vi "DETECTION REPORT for manual.vi"(7 "NEW PARAMETERS":T1, 8 "error in (no error)":errorcluster, 9 "return value 3":cluster{"major":dbl, "minor":dbl, "average":dbl}, 10 "Image File Path":path, 11 "Main Ref":T2) -> (0 "error out":errorcluster)   [LabVIEW 2025]
uses:
  <vilib>/Exaprom PDF/Controls/Font Controls/Font complete cluster.ctl
  <vilib>/Exaprom PDF/Controls/Font Controls/Font size.ctl
  <vilib>/Exaprom PDF/Controls/Font Controls/Font color.ctl
  <vilib>/Exaprom PDF/Controls/Font Controls/Type and encoding.ctl
  <vilib>/Exaprom PDF/Controls/Text Controls/Unicode/Type and run direction.ctl
  <vilib>/Exaprom PDF/Controls/Header, Footer and Watermark Controls/Header or Footer  Text cluster.ctl
  <vilib>/Exaprom PDF/Controls/Table Controls/Cell Alignment 20px.ctl
  <vilib>/Exaprom PDF/Controls/Text Controls/Line spacing.ctl
  <vilib>/Exaprom PDF/Controls/Font Controls/Font complete cluster horizontal.ctl
  <vilib>/Exaprom PDF/Controls/Header, Footer and Watermark Controls/Header or Footer Line cluster.ctl
  <vilib>/Exaprom PDF/Controls/Header, Footer and Watermark Controls/Header Footer Line.ctl
  <vilib>/Exaprom PDF/Controls/Header, Footer and Watermark Controls/Watermark Text Cluster.ctl
  <vilib>/Exaprom PDF/Controls/Header, Footer and Watermark Controls/Watermark Position.ctl
  <vilib>/Exaprom PDF/Controls/Header, Footer and Watermark Controls/Header footer horiz alignment.ctl
  <vilib>/Exaprom PDF/Controls/Image Controls/Image alignment and position.ctl
  <vilib>/Exaprom PDF/Controls/Image Controls/Image aligment.ctl
  <vilib>/Exaprom PDF/Controls/Image Controls/Image border.ctl
  <vilib>/Exaprom PDF/Controls/Table Controls/Table properties.ctl
  <vilib>/Exaprom PDF/Controls/Table Controls/Table position.ctl
  <vilib>/Exaprom PDF/Controls/Header, Footer and Watermark Controls/Header or Footer.ctl
  <vilib>/Exaprom PDF/Controls/Header, Footer and Watermark Controls/Header or Footer  Image cluster.ctl
  <vilib>/Exaprom PDF/Controls/Table Controls/Cell Font, type, Alignment and LS V2.ctl
  <vilib>/Exaprom PDF/Controls/Table Controls/Cell Type, Alignment and LS.ctl
  <vilib>/Exaprom PDF/Controls/Table Controls/Text vertical arrangement.ctl
  <vilib>/Utility/error.llb/Trim Whitespace One-Sided.vi
  <vilib>/Exaprom PDF/VIs/Low level/Header, Footer and Watermark Low level/Append Image HF.vi
  <vilib>/Exaprom PDF/VIs/Low level/Header, Footer and Watermark Low level/Append Text HF.vi
  <vilib>/Exaprom PDF/VIs/Low level/Header, Footer and Watermark Low level/AppendLine seperator.vi
  <vilib>/Exaprom PDF/VIs/Text/Append Phrase.vi
  <vilib>/Exaprom PDF/VIs/Low level/Header, Footer and Watermark Low level/Append Watermark Text.vi
panel:
  in  "Watermark Text 2":T3={"Text "="PALTRO", "Opacity (%)"=5.0, "Position"={"Position"=enum."Center (text section)", "X"=0.0, "Y"=0.0}, "Automatic"=TRUE, "Font"={"Font Name"="", "Size"=-1.0, "Color"=0}, "Alignment"=enum."Center", "Rotate(°)"=0.0}
  in  "Footer Line 2":T8={"H/F Line"=enum."Horizontal line", "Thickness (point)"=0.75, " Colour"=7171459}
  in  "Header Line":T8={"H/F Line"=enum."Horizontal line", "Thickness (point)"=0.75, " Colour"=7171459}
  in  "Footer Text":T10={"Start at page"=1, "Cell Alignment"=4, "Line spacing"=enum."Select", "Text"="Fully automated next-gen fuel and lubricant testers: BOCLE-adv , HFRR-ADV , FBT-3-P", "Font complete"={"Name"="", "Size"=5.0, "Color"=16777224, "Style"={"Bold"=FALSE, "Italic"=FALSE, "Underline"=TRUE, "Strikeout"=FALSE}, "Type"={"Type&direction"=enum."Select", "Embedded"=FALSE, "Encoding"=""}}, "Link"="https://www.paltro.com/products/product-selector/lubricity"}
  in  "Date and Time :":string
  in  "Observations :":string
  in  "Scar Image Path :":path
  in  "Header or footer":T10={"Start at page"=1, "Cell Alignment"=4, "Line spacing"=enum."Select", "Text"="                                            ", "Font complete"={"Name"="", "Size"=-1.0, "Color"=0, "Style"={"Bold"=FALSE, "Italic"=FALSE, "Underline"=FALSE, "Strikeout"=FALSE}, "Type"={"Type&direction"=enum."Select", "Embedded"=FALSE, "Encoding"=""}}, "Link"=""}
  in  "Font":T16={"Name"="", "Size"=18.0, "Color"=0, "Style"={"Bold"=TRUE, "Italic"=FALSE, "Underline"=FALSE, "Strikeout"=FALSE}, "Type"={"Type&direction"=enum."Select", "Embedded"=FALSE, "Encoding"=""}}
  in  "Font 2":T16={"Name"="", "Size"=6.0, "Color"=0, "Style"={"Bold"=FALSE, "Italic"=TRUE, "Underline"=FALSE, "Strikeout"=FALSE}, "Type"={"Type&direction"=enum."Select", "Embedded"=FALSE, "Encoding"=""}}
  in  "File Name :":string(combo)
  out "folder names":string[](array[string])
  out "path out":path
  in  "Automated":bool
  in  "Test Method":string
  in  "Fuel Description":string
  out "Operator :":string
types:
  T1 = cluster{"Initial Humidity (%RH)":string, "Final Humidity (%RH)":string, "Initial Air Temperature (°C)":string, "Final Air Temperature (°C)":string, "Specimen Tested":string, "Remarks":string}
  T2 = cluster{"File Name":string, "Test Method":string, "Operator":string, "Fuel Description":string, "Date and time":string}
  T3 = typedef "Watermark Text Cluster.ctl" = cluster{"Text ":string, "Opacity (%)":sgl, "Position":cluster{"Position":T4, "X":sgl, "Y":sgl}, "Automatic":bool, "Font":cluster{"Font Name":string, "Size":T5, "Color":T6}, "Alignment":T7, "Rotate(°)":sgl}
  T4 = typedef "Watermark Position.ctl" = enum16{"Absolute", "Center (page)", "Center (text section)"}
  T5 = typedef "Font size.ctl" = sgl
  T6 = typedef "Font color.ctl" = u32
  T7 = typedef "Header footer horiz alignment.ctl" = enum16{"Left", "Center", "Right"}
  T8 = typedef "Header or Footer Line cluster.ctl" = cluster{"H/F Line":T9, "Thickness (point)":sgl, " Colour":u32}
  T9 = typedef "Header Footer Line.ctl" = enum16{"No line", "Horizontal line"}
  T10 = typedef "Header or Footer  Text cluster.ctl" = cluster{"Start at page":i32, "Cell Alignment":T11, "Line spacing":T12, "Text":string, "Font complete":T13, "Link":string}
  T11 = typedef "Cell Alignment 20px.ctl" = u16
  T12 = typedef "Line spacing.ctl" = enum16{"Select", "1.0", "1.5", "2.0"}
  T13 = typedef "Font complete cluster horizontal.ctl" = cluster{"Name":string, "Size":T5, "Color":T6, "Style":cluster{"Bold":bool, "Italic":bool, "Underline":bool, "Strikeout":bool}, "Type":T14}
  T14 = typedef "Type and encoding.ctl" = cluster{"Type&direction":T15, "Embedded":bool, "Encoding":string}
  T15 = typedef "Type and run direction.ctl" = enum16{"Select", "ASCII", "UTF-16", "UTF-16 (default)", "UTF-16 (LTR)", "UTF-16 (RTL)"}
  T16 = typedef "Font complete cluster.ctl" = cluster{"Name":string, "Size":T5, "Color":T6, "Style":cluster{"Bold":bool, "Italic":bool, "Underline":bool, "Strikeout":bool}, "Type":T14}
  T17 = typedef "Cell Font, type, Alignment and LS V2.ctl" = cluster{"Cell Type, Alignment and LS":T18, "Font":T16}
  T18 = typedef "Cell Type, Alignment and LS.ctl" = cluster{"Cell Alignment":T11, "Text rotation":T19, "Line spacing":T12}
  T19 = typedef "Text vertical arrangement.ctl" = enum16{"None", "Clockwise", "Counterclockwise"}
  T20 = typedef "Header or Footer  Image cluster.ctl" = cluster{"Start at page":i32, "Cell Alignment":T11, "Path":path, "Image (%)":sgl, "Link":string}
  T21 = typedef "Image alignment and position.ctl" = cluster{"Alignment":T22, "X ":sgl, "Y":sgl, "Indentation":sgl}
  T22 = typedef "Image aligment.ctl" = enum16{"Absolute (X,Y)", "Left", "Center", "Right", "Left (textwrap)", "Right (textwrap)"}
  T23 = typedef "Image border.ctl" = cluster{"Show?":bool, "Thickness (point)":sgl, "Color":u32}
  T24 = typedef "Table properties.ctl" = cluster{"Table position":T25, "SpacingBefore (points)":sgl, "SpacingAfter (points)":sgl}
  T25 = typedef "Table position.ctl" = i32
  T26 = typedef "Header or Footer.ctl" = enum16{"Header", "Footer"}
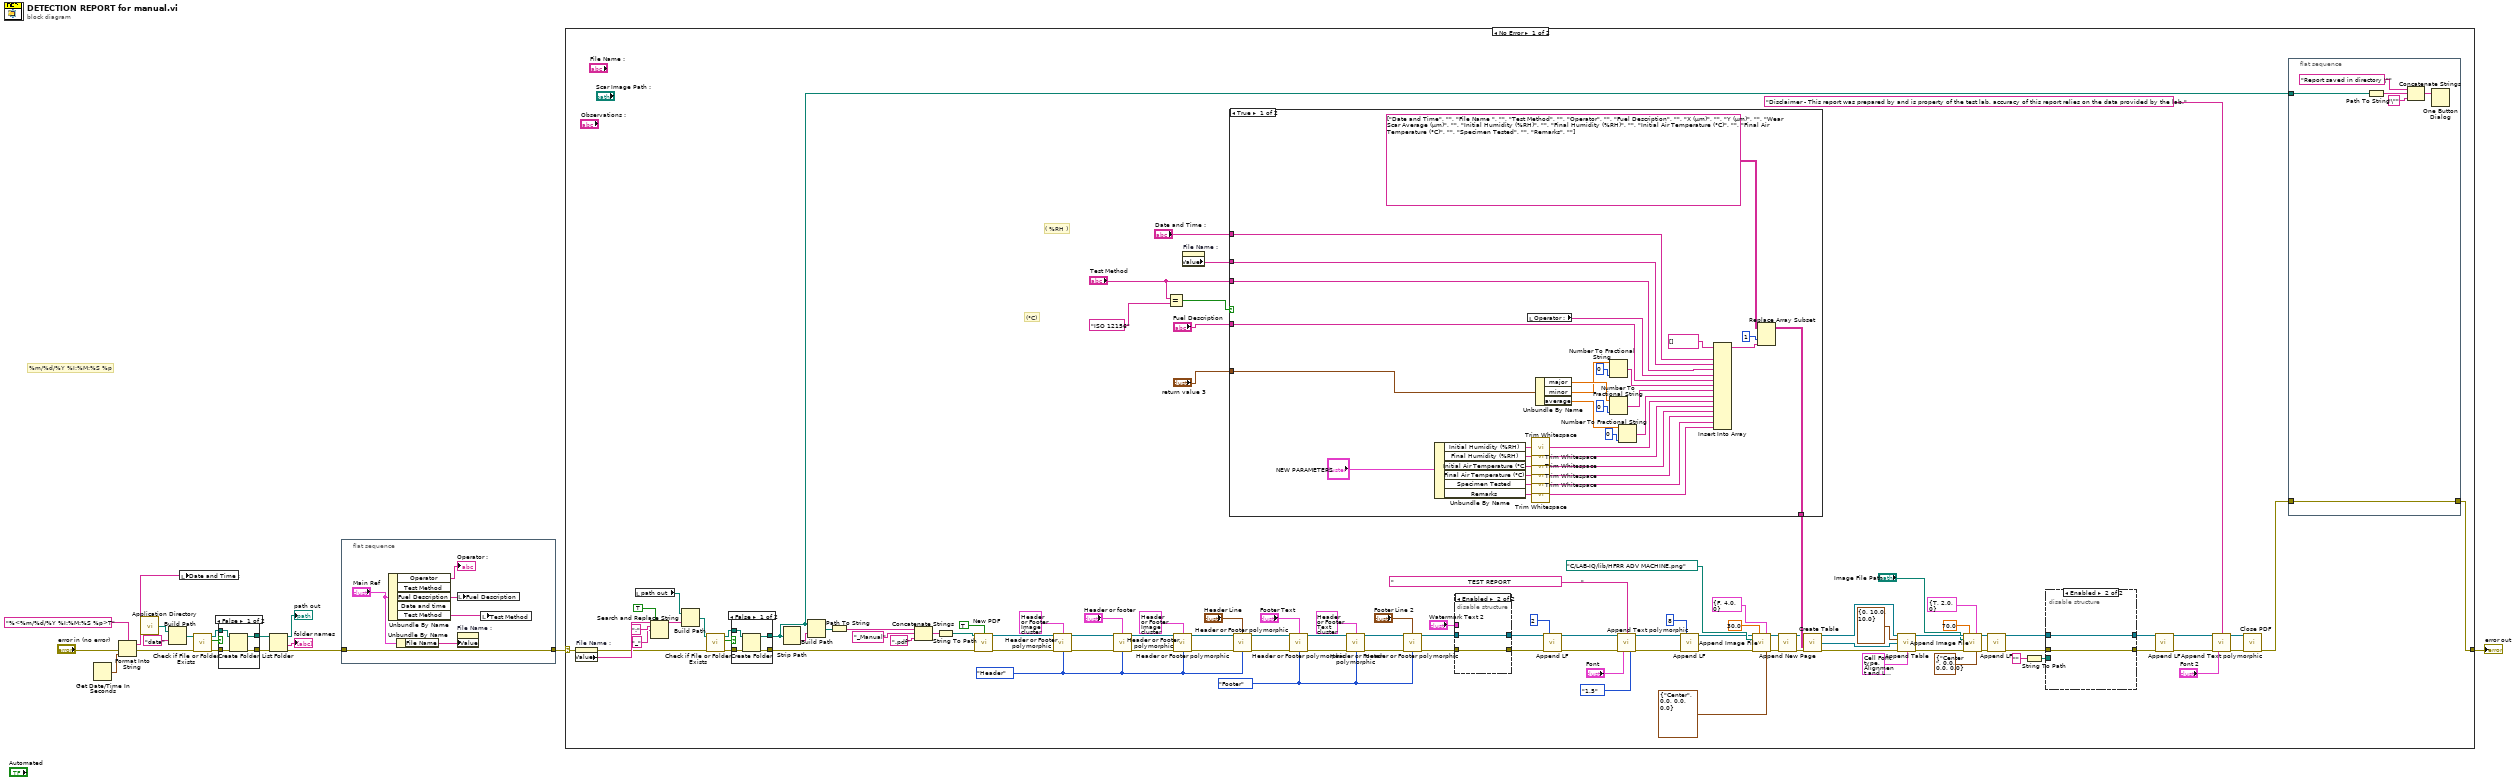
[diagram p0: block diagram]
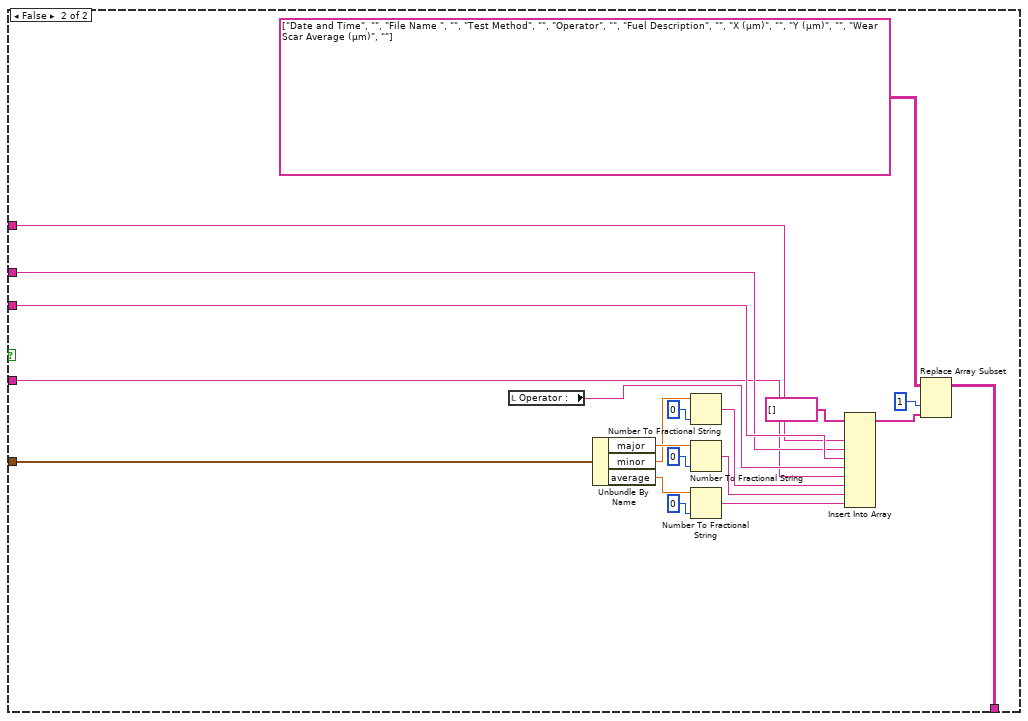
[diagram p2: hidden frame]
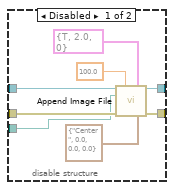
[diagram p3: hidden frame]
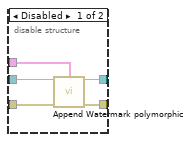
[diagram p4: hidden frame]
diagram:
  # "%m/%d/%Y %I:%M:%S %p"
  n1 = Get Date/Time In Seconds() -> (seconds since 1Jan1904=w7:timestamp)
  n2 = Format Into String(format string="%<%m/%d/%Y %I:%M:%S %p>T", error in="error in (no error)", w7) -> (resulting string=w1:string, error out=w5:errorcluster)  [unwired: 1 in]
  n3 = call <vilib>:"Application Directory.vi"() -> ("Application Directory"=w9:path)
  n4 = Build Path(base path=w9, name or relative path="data") -> (appended path=w8:path)
  n5 = local write "Date and Time :"(w1) -> ()
  n6 = call <vilib>:"Check if File or Folder Exists.vi"("error in (no error)"=w5, "path"=w8) -> ("error out"=w13:errorcluster, "file or folder exists?"=w15:bool, "dup path"=w14:path)  [unwired: 7 in]
  n7 = case shown="False" w15 {
    tunnel: w14 -> [w22 w23]
    tunnel: w13 -> [w21 w24]
    tunnel: [w20 w24] -> w18
    tunnel: [w19 w23] -> w16
    frame False {
      n8 = Create Folder(path (use dialog)=w22, error in=w21) -> (created path=w19:path, error out=w20:errorcluster)  [unwired: 1 in, 1 out]
    }
    frame True {
    }
  }
  n9 = List Folder(path=w16, error in=w18) -> (path out=→"path out":path, folder names=→"folder names":string[], error out=w3:errorcluster)  [unwired: 2 in, 1 out]
  n10 = flat-sequence {
    tunnel: w3 -> [w26]
    tunnel: [w26] -> w2
    frame #0 {
      n11 = Unbundle By Name("Main Ref") -> ("Operator"=→"Operator :":string, "Fuel Description"=w27:string, "Test Method"=w25:string)  [unwired: 2 out]
      n12 = Unbundle By Name("Main Ref") -> ("File Name"=w30:string)
      n13 = local write "Fuel Description"(w27) -> ()
      n14 = property on="File Name :" class="CmbBox"("Value"=w30) -> ()  [unwired: 2 in, 2 out]
      n15 = local write "Test Method"(w25) -> ()
    }
  }
  n16 = case shown="No Error" w2 {
    selector: w2 -> [w51 _]
    tunnel: [w50 _] -> w11
    frame No Error {
      w63 = Header_or_Footer."Header" ("Position")
      w92 = Header_or_Footer."Footer" ("Position")
      # "( %RH )"
      # "(°C)"
      n17 = property on="File Name :" class="CmbBox"(error in=w51) -> (error out=w52:errorcluster, "Value"=w53:string)  [unwired: 1 in, 1 out]
      n18 = local read "path out"() -> (w54:path)
      n19 = Search and Replace String(replace all?=TRUE ("replace all? (F)"), input string=w53, search string=":", replace string="_" ("replace string (\"\")")) -> (result string=w82:string)  [unwired: 4 in, 3 out]
      n20 = Build Path(base path=w54, name or relative path=w82) -> (appended path=w106:path)
      n21 = call <vilib>:"Check if File or Folder Exists.vi"("error in (no error)"=w52, "path"=w106) -> ("error out"=w103:errorcluster, "file or folder exists?"=w105:bool, "dup path"=w104:path)  [unwired: 7 in]
      n22 = case shown="False" w105 {
        tunnel: w104 -> [w214 w215]
        tunnel: w103 -> [w213 w216]
        tunnel: [w212 w216] -> w102
        tunnel: [w211 w215] -> w55
        frame False {
          n23 = Create Folder(path (use dialog)=w214, error in=w213) -> (created path=w211:path, error out=w212:errorcluster)  [unwired: 1 in, 1 out]
        }
        frame True {
        }
      }
      n24 = Strip Path(path=w55) -> (name=w108:string)  [unwired: 1 out]
      n25 = Build Path(base path=w55, name or relative path=w108) -> (appended path=w107:path)
      n26 = Path To String(path=w107) -> (string=w49:string)
      n27 = Concatenate Strings(w49, "_Manual" ("string"), ".pdf" ("string")) -> (w109:string)
      n28 = String To Path(string=w109) -> (path=w101:path)
      n29 = call <vilib>:"New PDF.vi"("PDF Path"=w101, "Overwrite?"=TRUE, "error in (no error)"=w102) -> ("PDF Report"=w123:refnum<class "PDF Report Class.lvclass">, "error out"=w124:errorcluster)  [unwired: 11 in]
      n30 = call-poly <vilib>:"Header or Footer polymorphic.vi"("PDF Report IN"=w123, "Header or footer"=T20 {"Start at page"=1, "Cell Alignment"=4, "Path"=path "C:/LAB-IQ/lib/paltro logo.png", "Image (%)"=100.0, "Link"="https://www.paltro.com/"} ("HEADER Image"), "error in (no error)"=w124, "Position"=w63) -> ("PDF Report OUT"=w80:refnum<class "PDF Report Class.lvclass">, "error out"=w81:errorcluster)  [unwired: 10 out]
      n31 = call-poly <vilib>:"Header or Footer polymorphic.vi"("PDF Report IN"=w80, "Header or footer"="Header or footer", "error in (no error)"=w81, "Position"=w63) -> ("PDF Report OUT"=w78:refnum<class "PDF Report Class.lvclass">, "error out"=w79:errorcluster)  [unwired: 10 out]
      n32 = Equal?(x="Test Method", y="ISO 12156") -> (x = y?=w31:bool)
      n33 = call-poly <vilib>:"Header or Footer polymorphic.vi"("PDF Report IN"=w78, "Header or footer"=T20 {"Start at page"=1, "Cell Alignment"=6, "Path"=path "C:/LAB-IQ/lib/HFRR_adv.png", "Image (%)"=30.0, "Link"="https://www.paltro.com/products/test-and-measurement/bocle--automated-ball-on-cylinder-lubricity-evaluator"} ("HEADER Image  2"), "error in (no error)"=w79, "Position"=w63) -> ("PDF Report OUT"=w95:refnum<class "PDF Report Class.lvclass">, "error out"=w96:errorcluster)  [unwired: 10 out]
      n34 = property on="File Name :" class="CmbBox"() -> ("Value"=w35:string)  [unwired: 2 in, 2 out]
      n35 = case shown="True" w31 {
        tunnel: [w167 w187] -> w131
        tunnel: "Test Method" -> [w146 w172]
        tunnel: "Date and Time :" -> [w145 w171]
        tunnel: w35 -> [w144 w170]
        tunnel: "Fuel Description" -> [w143 w169]
        tunnel: "return value 3" -> [w142 w168]
        frame True {
          n36 = Unbundle By Name("NEW PARAMETERS") -> ("Initial Humidity (%RH)"=w152:string, "Final Humidity (%RH)"=w151:string, "Initial Air Temperature (°C)"=w150:string, "Final Air Temperature (°C)"=w149:string, "Specimen Tested"=w148:string, "Remarks"=w147:string)
          n37 = local read "Operator :"() -> (w153:string)
          n38 = call <vilib>:"Trim Whitespace.vi"("string"=w152) -> ("trimmed string"=w140:string)  [unwired: 1 in]
          n39 = call <vilib>:"Trim Whitespace.vi"("string"=w151) -> ("trimmed string"=w139:string)  [unwired: 1 in]
          n40 = call <vilib>:"Trim Whitespace.vi"("string"=w150) -> ("trimmed string"=w138:string)  [unwired: 1 in]
          n41 = call <vilib>:"Trim Whitespace.vi"("string"=w149) -> ("trimmed string"=w137:string)  [unwired: 1 in]
          n42 = call <vilib>:"Trim Whitespace.vi"("string"=w148) -> ("trimmed string"=w136:string)  [unwired: 1 in]
          n43 = call <vilib>:"Trim Whitespace.vi"("string"=w147) -> ("trimmed string"=w135:string)  [unwired: 1 in]
          n44 = Unbundle By Name(w142) -> ("major"=w156:dbl, "minor"=w155:dbl, "average"=w154:dbl)
          n45 = Number To Fractional String(number=w155, precision (6)=i16 0) -> (F-format string=w157:string)  [unwired: 2 in]
          n46 = Number To Fractional String(number=w156, precision (6)=i16 0) -> (F-format string=w158:string)  [unwired: 2 in]
          n47 = Number To Fractional String(number=w154, precision (6)=i16 0) -> (F-format string=w159:string)  [unwired: 2 in]
          n48 = Insert Into Array(array=string[] [], new element #1=w145, new element #2=w144, new element #3=w146, new element #4=w153, new element #5=w143, new element #6=w157, new element #7=w158, new element #8=w159, new element #9=w140, new element #10=w139, new element #11=w138, new element #12=w137, new element #13=w136, new element #14=w135) -> (w166:string[])  [unwired: 1 in]
          n49 = Replace Array Subset(array=string[][] [["Date and Time", ""], ["File Name ", ""], ["Test Method", ""], ["Operator", ""], ["Fuel Description", ""], ["X (µm)", ""], ["Y (µm)", ""], ["Wear Scar Average (µm)", ""], ["Initial Humidity (%RH)", ""], ["Final Humidity (%RH)", ""], ["Initial Air Temperature (°C)", ""], ["Final Air Temperature (°C)", ""], ["Specimen Tested", ""], ["Remarks", ""]] ("Text Data 2D [ ]"), new element=w166, index (col)=1 ("disabled index (col)")) -> (w167:string[][])  [unwired: 1 in]
        }
        frame False {
          n50 = local read "Operator :"() -> (w173:string)
          n51 = Unbundle By Name(w168) -> ("major"=w176:dbl, "minor"=w175:dbl, "average"=w174:dbl)
          n52 = Number To Fractional String(number=w175, precision (6)=i16 0) -> (F-format string=w177:string)  [unwired: 2 in]
          n53 = Number To Fractional String(number=w176, precision (6)=i16 0) -> (F-format string=w178:string)  [unwired: 2 in]
          n54 = Number To Fractional String(number=w174, precision (6)=i16 0) -> (F-format string=w179:string)  [unwired: 2 in]
          n55 = Insert Into Array(array=string[] [], new element #1=w171, new element #2=w170, new element #3=w172, new element #4=w173, new element #5=w169, new element #6=w177, new element #7=w178, new element #8=w179) -> (w186:string[])  [unwired: 1 in]
          n56 = Replace Array Subset(array=string[][] [["Date and Time", ""], ["File Name ", ""], ["Test Method", ""], ["Operator", ""], ["Fuel Description", ""], ["X (µm)", ""], ["Y (µm)", ""], ["Wear Scar Average (µm)", ""]] ("Text Data 2D [ ]"), new element=w186, index (col)=1 ("disabled index (col)")) -> (w187:string[][])  [unwired: 1 in]
        }
      }
      n57 = call-poly <vilib>:"Header or Footer polymorphic.vi"("PDF Report IN"=w95, "H/F Line"="Header Line", "error in (no error)"=w96, "Position"=w63) -> ("PDF Report OUT"=w127:refnum<class "PDF Report Class.lvclass">, "error out"=w126:errorcluster)  [unwired: 1 in, 9 out]
      n58 = call-poly <vilib>:"Header or Footer polymorphic.vi"("PDF Report IN"=w127, "Header or footer"="Footer Text", "error in (no error)"=w126, "Position"=w92) -> ("PDF Report OUT"=w129:refnum<class "PDF Report Class.lvclass">, "error out"=w128:errorcluster)  [unwired: 10 out]
      n59 = call-poly <vilib>:"Header or Footer polymorphic.vi"("PDF Report IN"=w129, "Header or footer"=T10 {"Start at page"=1, "Cell Alignment"=6, "Line spacing"=enum."Select", "Text"="www.paltro.com", "Font complete"={"Name"="", "Size"=6.0, "Color"=16777224, "Style"={"Bold"=FALSE, "Italic"=FALSE, "Underline"=TRUE, "Strikeout"=FALSE}, "Type"={"Type&direction"=enum."Select", "Embedded"=FALSE, "Encoding"=""}}, "Link"="https://www.paltro.com/"} ("Footer Text 2"), "error in (no error)"=w128, "Position"=w92) -> ("PDF Report OUT"=w122:refnum<class "PDF Report Class.lvclass">, "error out"=w121:errorcluster)  [unwired: 10 out]
      n60 = call-poly <vilib>:"Header or Footer polymorphic.vi"("PDF Report IN"=w122, "H/F Line"="Footer Line 2", "error in (no error)"=w121, "Position"=w92) -> ("PDF Report OUT"=w115:refnum<class "PDF Report Class.lvclass">, "error out"=w116:errorcluster)  [unwired: 1 in, 9 out]
      n61 = disable-structure shown="Enabled" {
        disable-tunnel: "Watermark Text 2" -> [w208 _]
        disable-tunnel: w116 -> [w207 w210]
        disable-tunnel: w115 -> [w206 w209]
        disable-tunnel: [w205 w210] -> w74
        disable-tunnel: [w204 w209] -> w73
        frame Disabled {
          n62 = call-poly <vilib>:"Append Watermark polymorphic.vi"("PDF Report IN"=w206, "Watermark Text"=w208, "error in (no error)"=w207) -> ("PDF Report OUT"=w204:refnum<class "PDF Report Class.lvclass">, "error out"=w205:errorcluster)  [unwired: 1 in, 10 out]
        }
        frame Enabled {
        }
      }
      n63 = call <vilib>:"Append LF.vi"("PDF Report IN"=w73, "Number of LF (default 1)"=u8 2, "error in (no error)"=w74) -> ("PDF Report duplicate"=w71:refnum<class "PDF Report Class.lvclass">, "error out"=w72:errorcluster)  [unwired: 11 in]
      n64 = call-poly <vilib>:"Append Text polymorphic.vi"("PDF Report IN"=w71, "Text"="                                     TEST REPORT                                   ", "error in (no error)"=w72, "Font"="Font", "Line spacing"=Line_spacing."1.5") -> ("PDF Report OUT"=w59:refnum<class "PDF Report Class.lvclass">, "error out"=w60:errorcluster)  [unwired: 9 in]
      n65 = call <vilib>:"Append LF.vi"("PDF Report IN"=w59, "Number of LF (default 1)"=u8 8, "error in (no error)"=w60) -> ("PDF Report duplicate"=w62:refnum<class "PDF Report Class.lvclass">, "error out"=w61:errorcluster)  [unwired: 11 in]
      n66 = call <vilib>:"Append Image File.vi"("PDF Report IN"=w62, "Scale (%)"=sgl 30.0, "Border"=T23 {"Show?"=FALSE, "Thickness (point)"=4.0, "Color"=0}, "Image path"=path "C:/LAB-IQ/lib/HFRR ADV MACHINE.png", "error in (no error)"=w61, "Position and indentation"=T21 {"Alignment"=enum."Center", "X "=0.0, "Y"=0.0, "Indentation"=0.0}) -> ("PDF Report OUT"=w99:refnum<class "PDF Report Class.lvclass">, "error out"=w100:errorcluster)  [unwired: 6 in, 2 out]
      n67 = call <vilib>:"Append New Page.vi"("PDF Report"=w99, "error in (no error)"=w100) -> ("PDF Report duplicate"=w97:refnum<class "PDF Report Class.lvclass">, "error OUT"=w98:errorcluster)  [unwired: 12 in]
      n68 = call <vilib>:"Create Table.vi"("PDF Report IN"=w97, "Text Data 2D [ ]"=w131, "error in (no error)"=w98) -> ("PDF Report duplicate"=w112:refnum<class "PDF Report Class.lvclass">, "PDF Table"=w114:refnum<class "Pdfp Table Class.lvclass">, "error out"=w110:errorcluster)  [unwired: 10 in]
      n69 = call <vilib>:"Append Table.vi"("PDF Report IN"=w112, "Table properties"=T24 {"Table position"=0, "SpacingBefore (points)"=10.0, "SpacingAfter (points)"=10.0} ("Table properties  - Tables 2 to 4"), "PDF Table"=w114, "error in (no error)"=w110, "Datas format"=T17 {"Cell Type, Alignment and LS"={"Cell Alignment"=4, "Text rotation"=enum."None", "Line spacing"=enum."Select"}, "Font"={"Name"="", "Size"=-1.0, "Color"=0, "Style"={"Bold"=FALSE, "Italic"=FALSE, "Underline"=FALSE, "Strikeout"=FALSE}, "Type"={"Type&direction"=enum."Select", "Embedded"=FALSE, "Encoding"=""}}}) -> ("PDF Report OUT"=w113:refnum<class "PDF Report Class.lvclass">, "error out"=w111:errorcluster)  [unwired: 7 in, 2 out]
      n70 = call <vilib>:"Append Image File.vi"("PDF Report IN"=w113, "Scale (%)"=sgl 70.0, "Border"=T23 {"Show?"=TRUE, "Thickness (point)"=2.0, "Color"=0}, "Image path"="Image File Path", "error in (no error)"=w111, "Position and indentation"=T21 {"Alignment"=enum."Center", "X "=0.0, "Y"=0.0, "Indentation"=0.0}) -> ("PDF Report OUT"=w65:refnum<class "PDF Report Class.lvclass">, "error out"=w66:errorcluster)  [unwired: 6 in, 2 out]
      n71 = call <vilib>:"Append LF.vi"("PDF Report IN"=w65, "error in (no error)"=w66) -> ("PDF Report duplicate"=w43:refnum<class "PDF Report Class.lvclass">, "error out"=w44:errorcluster)  [unwired: 12 in]
      n72 = String To Path(string="") -> (path=w40:path)
      n73 = disable-structure shown="Enabled" {
        disable-tunnel: [w195 w197] -> w46
        disable-tunnel: [w194 w196] -> w45
        disable-tunnel: w44 -> [w191 w196]
        disable-tunnel: w43 -> [w190 w197]
        disable-tunnel: w40 -> [w188 _]
        frame Disabled {
          n74 = call <vilib>:"Append Image File.vi"("PDF Report IN"=w190, "Scale (%)"=sgl 100.0, "Border"=T23 {"Show?"=TRUE, "Thickness (point)"=2.0, "Color"=0}, "Image path"=w188, "error in (no error)"=w191, "Position and indentation"=T21 {"Alignment"=enum."Center", "X "=0.0, "Y"=0.0, "Indentation"=0.0}) -> ("PDF Report OUT"=w195:refnum<class "PDF Report Class.lvclass">, "error out"=w194:errorcluster)  [unwired: 6 in, 2 out]
        }
        frame Enabled {
        }
      }
      n75 = call <vilib>:"Append LF.vi"("PDF Report IN"=w46, "error in (no error)"=w45) -> ("PDF Report duplicate"=w41:refnum<class "PDF Report Class.lvclass">, "error out"=w42:errorcluster)  [unwired: 12 in]
      n76 = call-poly <vilib>:"Append Text polymorphic.vi"("PDF Report IN"=w41, "Text"="Disclaimer - This report was prepared by and is property of the test lab, accuracy of this report relies on the data provided by the lab.", "error in (no error)"=w42, "Font"="Font 2") -> ("PDF Report OUT"=w68:refnum<class "PDF Report Class.lvclass">, "error out"=w69:errorcluster)  [unwired: 10 in]
      n77 = call <vilib>:"Close PDF.vi"("PDF Report"=w68, "error in (no error)"=w69) -> ("error out"=w56:errorcluster)  [unwired: 12 in, 1 out]
      n78 = flat-sequence {
        tunnel: w56 -> [w203]
        tunnel: [w203] -> w50
        tunnel: w55 -> [w202]
        frame #0 {
          n79 = Path To String(path=w202) -> (string=w201:string)
          n80 = Concatenate Strings("Report saved in directory \"", w201, "\"" ("string")) -> (w198:string)
          n81 = One Button Dialog(message=w198) -> ()  [unwired: 1 in, 1 out]
        }
      }
    }
    frame Error {
      # "WHEN USER PRESSED CLOSE BUTTON"
    }
  }
  "error out" <- w11
